vi "ReadDAQConfig.vi"(8 "error in":errorcluster caption="错误输入", 11 "产品型号":refnum<vi>) -> (0 "error out":errorcluster caption="错误输出", 3 "DAQConfig":T1={"DO"=[["ACC", "Dev1/port2/line0", "Dev1/port0/line24"], ["ILL", "Dev1/port2/line1", "Dev1/port0/line25"], ["BACK", "Dev1/port2/line2", "Dev1/port0/line26"], ["BRAKE", "Dev1/port2/line3", "Dev1/port0/line27"], ["PowerON_Vps", "Dev1/port2/line4", "Dev1/port0/line28"], ["PowerON_+B", "Dev1/port2/line5", "Dev1/port0/line29"], ["SW", "Dev1/port2/line6", "Dev1/port0/line30"], ["SW1", "Dev1/port0/line5", "Dev1/port0/line13"], ["SW2", "Dev1/port0/line6", "Dev1/port0/line14"], ["LineOut1", "Dev1/port1/line3", "Dev1/port0/line19"], ["LineOut2", "Dev1/port1/line2", "Dev1/port0/line18"], ["LineOut3", "Dev1/port1/line5", "Dev1/port0/line21"], ["LineOut4", "Dev1/port1/line4", "Dev1/port0/line20"], ["LineOut5", "Dev1/port1/line7", "Dev1/port0/line23"], ["LineOut6", "Dev1/port1/line6", "Dev1/port0/line22"], ["SPK", "Dev1/port2/line7", "Dev1/port0/line31"], ["SPK2", "Dev1/port0/line7", "Dev1/port0/line15"], ["IPOD_DET", "Dev1/port1/line0", "Dev1/port0/line16"], ["RING", "Dev1/port1/line1", "Dev1/port0/line17"], ["PASSButton", "Dev1/port0/line2", "Dev1/port0/line10"], ["FAILButton", "Dev1/port0/line3", "Dev1/port0/line11"], ["DO_IPOD+5V", "Dev1/port0/line4", "Dev1/port0/line12"]], "DI"=[["PowerSimulate", "Dev1/ao0", "Dev1/ao2"], ["AudioSW", "Dev1/ao1", "Dev1/ao3"]]})   [LabVIEW 2013]
uses:
  Ctl/IOConfig.ctl
  <vilib>/Utility/NIReport.llb/NI_report.lvclass
  GlobValue.vi
  <vilib>/addons/_office/excel.llb/Excel Get Data ([str]).vi
  <vilib>/addons/_office/NI_ReportGenerationToolkit.lvlib
  <vilib>/Utility/NIReport.llb/Excel/NI_Excel.lvclass
panel:
  out "DI":string[][](table)=[["PowerMonitor", "Dev1/ai5", "Dev1/ai21"], ["FL", "Dev1/ai0", "Dev1/ai16"], ["FR", "Dev1/ai1", "Dev1/ai17"], ["RL", "Dev1/ai2", "Dev1/ai18"], ["RR", "Dev1/ai3", "Dev1/ai19"], ["FLOUT", "Dev1/ai6", "Dev1/ai22"], ["FROUT", "Dev1/ai7", "Dev1/ai23"], ["RLOUT", "Dev1/ai13", "Dev1/ai29"], ["RROUT", "Dev1/ai14", "Dev1/ai30"], ["SUB", "Dev1/ai15", "Dev1/ai31"], ["Current", "Dev1/ai4", "Dev1/ai20"], ["IPOD+5V", "Dev1/ai12", "Dev1/ai28"]]
  out "DO":string[][](table)=[["ACC", "Dev1/port2/line0", "Dev1/port0/line24"], ["ILL", "Dev1/port2/line1", "Dev1/port0/line25"], ["BACK", "Dev1/port2/line2", "Dev1/port0/line26"], ["BRAKE", "Dev1/port2/line3", "Dev1/port0/line27"], ["PowerON_Vps", "Dev1/port2/line4", "Dev1/port0/line28"], ["PowerON_+B", "Dev1/port2/line5", "Dev1/port0/line29"], ["SW", "Dev1/port2/line6", "Dev1/port0/line30"], ["SW1", "Dev1/port0/line5", "Dev1/port0/line13"], ["SW2", "Dev1/port0/line6", "Dev1/port0/line14"], ["LineOut1", "Dev1/port1/line3", "Dev1/port0/line19"], ["LineOut2", "Dev1/port1/line2", "Dev1/port0/line18"], ["LineOut3", "Dev1/port1/line5", "Dev1/port0/line21"], ["LineOut4", "Dev1/port1/line4", "Dev1/port0/line20"], ["LineOut5", "Dev1/port1/line7", "Dev1/port0/line23"], ["LineOut6", "Dev1/port1/line6", "Dev1/port0/line22"], ["SPK", "Dev1/port2/line7", "Dev1/port0/line31"], ["SPK2", "Dev1/port0/line7", "Dev1/port0/line15"], ["IPOD_DET", "Dev1/port1/line0", "Dev1/port0/line16"], ["RING", "Dev1/port1/line1", "Dev1/port0/line17"], ["PASSButton", "Dev1/port0/line2", "Dev1/port0/line10"], ["FAILButton", "Dev1/port0/line3", "Dev1/port0/line11"], ["DO_IPOD+5V", "Dev1/port0/line4", "Dev1/port0/line12"]]
  out "ConfigPath":string="D:\\导航\\AVN\\config\\DAQConfig.xls"
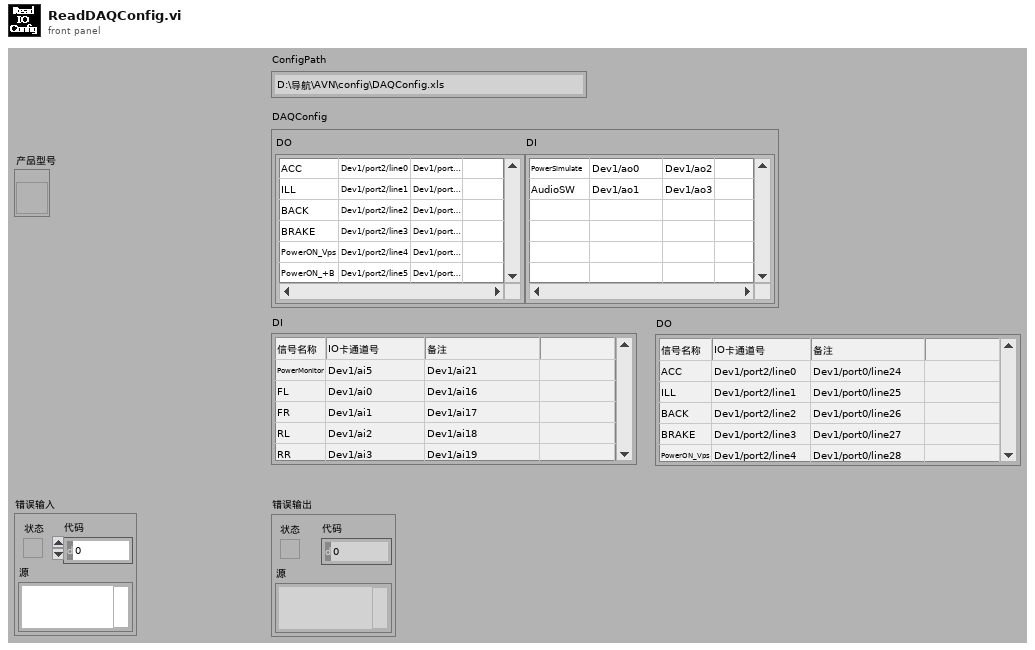
[diagram p1: front panel]
types:
  T1 = typedef "IOConfig.ctl" = cluster{"DO":string[][], "DI":string[][]}
  T2 = enum16{"maximized", "minimized", "normal", "no change"}
  T3 = enum16{"Standard Report", "HTML", "Word", "Excel"}
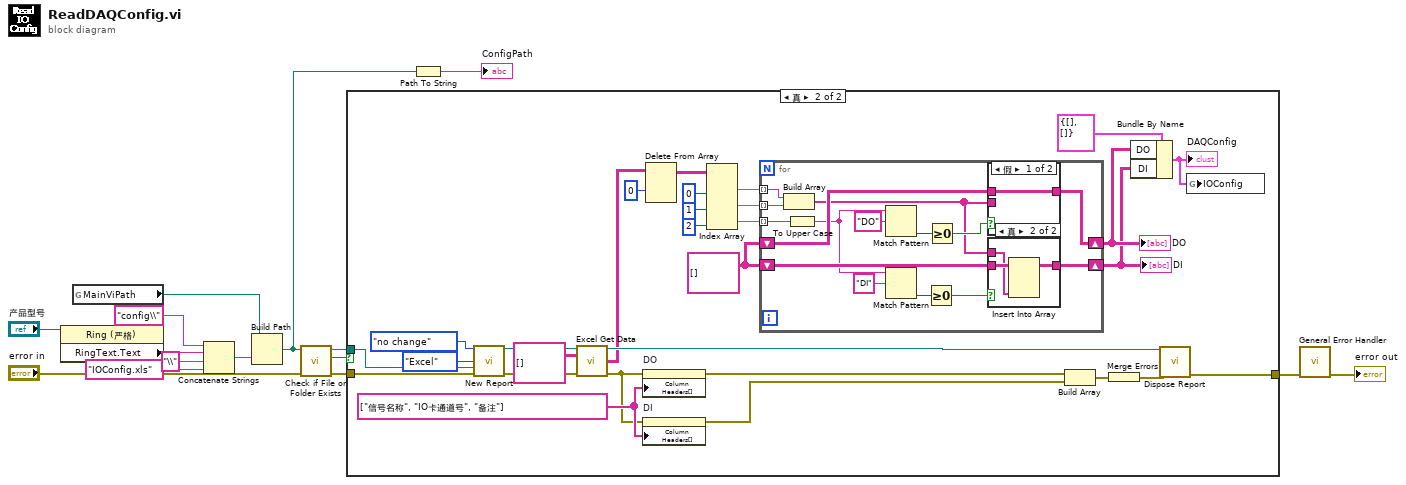
[diagram p0: block diagram]
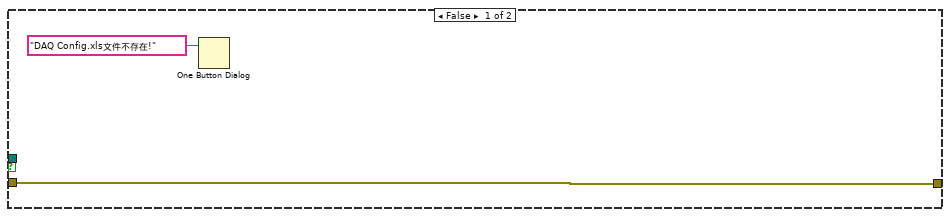
[diagram p2: hidden frame]
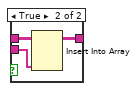
[diagram p3: hidden frame]
diagram:
  n1 = property on="属性节点" class="Ring (严格)"(reference="产品型号") -> ("RingText.Text"=w3:string)  [unwired: 1 in, 2 out]
  n2 = global read "GlobValue.vi" "MainViPath"() -> (w7:path)
  n3 = Concatenate Strings("config\\" ("连接的字符串"), w3, "\\" ("字符串"), "IOConfig.xls" ("连接的字符串")) -> (w1:string)
  n4 = Build Path(base path=w7, name or relative path=w1) -> (appended path=w12:path)
  n5 = call <vilib>:"Check if File or Folder Exists.vi"("error in (no error)"="error in", "path"=w12) -> ("error out"=w15:errorcluster, "file or folder exists?"=w14:bool, "dup path"=w9:path)  [unwired: 7 out]
  n6 = case shown="真" w14 {
    tunnel: w15 -> [w17 w45]
    tunnel: w9 -> [_ w46]
    tunnel: [w17 w43] -> w13
    frame False {
      n7 = One Button Dialog(message="DAQ Config.xls文件不存在!" ("消息")) -> ()  [unwired: 1 in, 1 out]
    }
    frame True {
      w22 = string[] ["信号名称", "IO卡通道号", "备注"]
      w28 = string[][] [] ("Array")
      n8 = call <vilib>:"New Report.vi"("window state (normal)"=T2."no change", "report type"=T3."Excel", "template (empty)"=w46, "error in (no error)"=w45) -> ("report out"=w38:refnum<class "NI_report.lvclass">, "error out"=w37:errorcluster)  [unwired: 2 in, 8 out]
      n9 = call-poly <vilib>:"Excel Get Data.vi"("report in"=w38, "data type"=string[][] [], "error in (no error)"=w37) -> ("report out"=w44:refnum<class "NI_report.lvclass">, "data"=w36:string[][], "error out"=w20:errorcluster)  [unwired: 10 in]
      n10 = property on="DO" class="Tbl (严格)"(error in=w20, "Column Headers[]"=w22) -> (error out=w27:errorcluster)  [unwired: 1 in, 1 out]
      n11 = property on="DI" class="Tbl (严格)"(error in=w20, "Column Headers[]"=w22) -> (error out=w21:errorcluster)  [unwired: 1 in, 1 out]
      n12 = Delete From Array(array=w36, index (row)=0 ("索引 (行)")) -> (array with subset deleted=w34:string[][])  [unwired: 2 in, 1 out]
      n13 = Index Array(array=w34, index (col) #1=0 ("禁用的索引 (列)"), index (col) #2=1 ("索引 (列)"), index (col) #3=2 ("索引 (列)")) -> (element #1=w32:string[], element #2=w26:string[], element #3=w24:string[])  [unwired: 3 in]
      n14 = for {
        shift-right: [w56] -> w19
        shift-left: w28 -> [w55]
        shift-right: [w60] -> w18
        shift-left: w28 -> [w59]
        tunnel: w32 -> [w52] mode=indexing
        tunnel: w26 -> [w51] mode=indexing
        tunnel: w24 -> [w47] mode=indexing
        n15 = Build Array(w52, w51) -> (w53:string[])
        n16 = To Upper Case(1:w47) -> (0:w54:string)
        n17 = Match Pattern(string=w54, regular expression="DO") -> (offset past match=w50:i32)  [unwired: 1 in, 3 out]
        n18 = Match Pattern(string=w54, regular expression="DI") -> (offset past match=w49:i32)  [unwired: 1 in, 3 out]
        n19 = Greater Or Equal To 0?(x=w49) -> (x >= 0?=w48:bool)
        n20 = Greater Or Equal To 0?(x=w50) -> (x >= 0?=w57:bool)
        n21 = case shown="假" w57 {
          tunnel: [w62 w64] -> w56
          tunnel: w55 -> [w62 w65]
          tunnel: w53 -> [_ w63]
          frame False {
          }
          frame True {
            n22 = Insert Into Array(array=w65, new element=w63) -> (w64:string[][])  [unwired: 2 in]
          }
        }
        n23 = case shown="真" w48 {
          tunnel: [w66 w68] -> w60
          tunnel: w59 -> [w66 w69]
          tunnel: w53 -> [_ w67]
          frame False {
          }
          frame True {
            n24 = Insert Into Array(array=w69, new element=w67) -> (w68:string[][])  [unwired: 2 in]
          }
        }
      }
      "DO" <- w19
      "DI" <- w18
      n25 = Build Array(w27, w21) -> (w41:errorcluster[])
      n26 = Merge Errors(w41) -> (w40:errorcluster)
      n27 = Bundle By Name(cluster=T1 {"DO"=[], "DI"=[]} ("DAQConfig"), "DO"=w19, "DI"=w18) -> (w23:T1)
      "DAQConfig" <- w23
      n28 = call-dynamic "Dispose Report.vi"("report in"=w44, "error in (no error)"=w40) -> ("error out"=w43:errorcluster)  [unwired: 3 in, 10 out]
      n29 = global write "GlobValue.vi" "IOConfig"(w23) -> ()
    }
  }
  n30 = Path To String(path=w12) -> (string=→"ConfigPath":string)
  n31 = call <vilib>:"General Error Handler.vi"("error in (no error)"=w13) -> ("error out"=→"error out":errorcluster)  [unwired: 10 in, 4 out]
